vi "c ctre phoenixpro Request Control BMS Manual Pwm Junction.vi"(4 "JunctionDutyCycle":dbl, 6 "JunctionSelect":i32, 7 "cancelOtherRequests":bool, 8 "error in (no error)":errorcluster, 9 "updateTime":dbl, 10 "ecuEncoding":u32, 11 "canbus":string) -> (0 "error out":errorcluster, 3 "function return":i32)   [LabVIEW 2020, in "CTRE_PhoenixTools.lvlib"]
doc: "CTREXPORT int c_ctre_phoenixpro_RequestControlBMSManualPwmJunction(const char *canbus, uint32_t ecuEncoding, double updateTime, bool cancelOtherRequests, int JunctionSelect, double JunctionDutyCycle);"
uses:
  <userlib>/CTRE_PhoenixTools/CTRE_PhoenixTools.lvlib
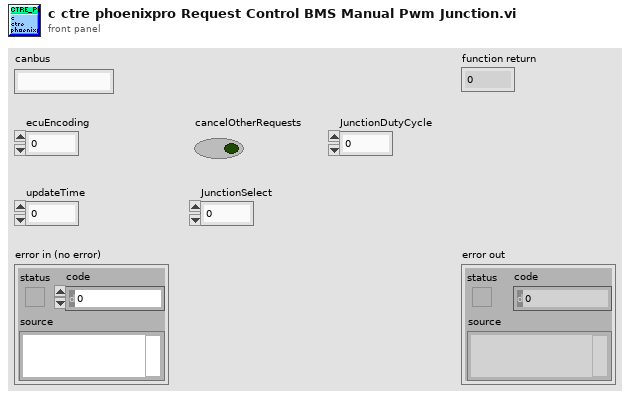
[diagram p1: front panel]
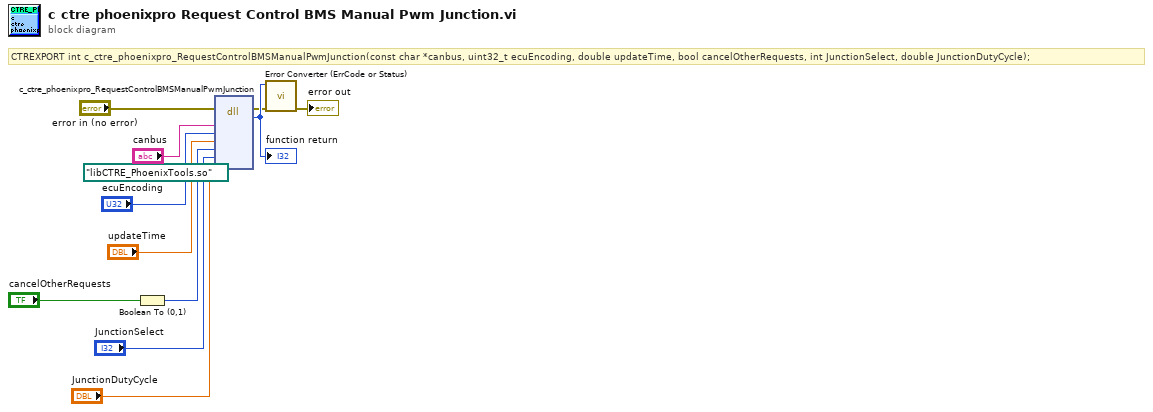
[diagram p0: block diagram]
diagram:
  # "CTREXPORT int c_ctre_phoenixpro_RequestControlBMSManualPwmJunction(const char *canbus, uint32_t ecuEncoding, double updateTime, bool cancelOtherRequests, int JunctionSelect, double JunctionDutyCycle);"
  n1 = Boolean To (0,1)(Boolean="cancelOtherRequests") -> (0, 1=w7:i16)
  n2 = dll-call lib="?" fn="c_ctre_phoenixpro_RequestControlBMSManualPwmJunction"(path in=path "libCTRE_PhoenixTools.so", error in="error in (no error)", "canbus"="canbus", "ecuEncoding"="ecuEncoding", "updateTime"="updateTime", "cancelOtherRequests"=w7, "JunctionSelect"="JunctionSelect", "JunctionDutyCycle"="JunctionDutyCycle") -> (error out=w3:errorcluster, "return type"=w12:i32)  [unwired: 7 in, 1 out]
  "function return" <- w12
  n3 = call <userlib>:"Error Converter (ErrCode or Status).vi"("error in (no error)"=w3, "error code"=w12) -> ("error out"=→"error out":errorcluster)  [unwired: 9 in]
